vi "Parse Policy.vi"(11 "Response body":string) -> (3 "Policy":T1)   [LabVIEW 2015, in "NI_AWS_IAM.lvlib"]
uses:
  NI_AWS_IAM.lvlib
  Policy.ctl
  XML Parsing/NI_XML Parsing.lvlib
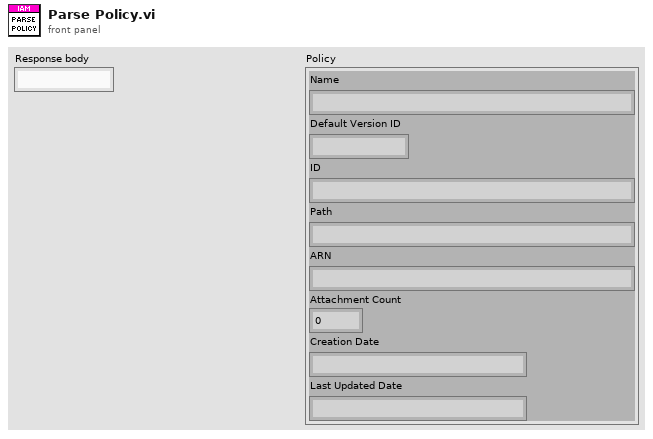
[diagram p1: front panel]
types:
  T1 = typedef "NI_AWS_IAM.lvlib/Policy.ctl" = cluster{"Name":string, "Default Version ID":string, "ID":string, "Path":string, "ARN":string, "Attachment Count":i32, "Creation Date":string, "Last Updated Date":string}
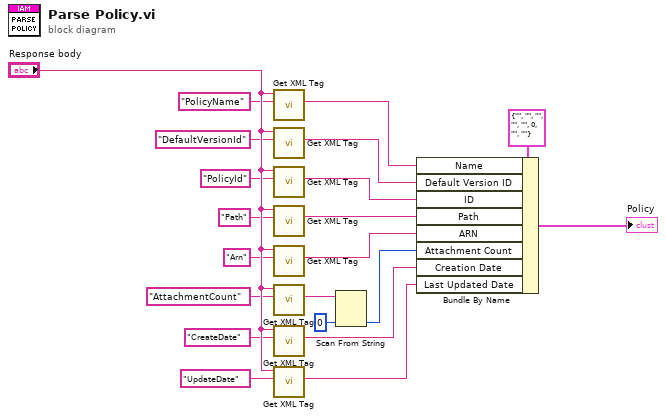
[diagram p0: block diagram]
diagram:
  n1 = call "Get XML Tag.vi"("Tag name"="PolicyName", "XML String in"="Response body") -> ("Tag value"=w10:string)  [unwired: 5 in, 4 out]
  n2 = call "Get XML Tag.vi"("Tag name"="DefaultVersionId", "XML String in"="Response body") -> ("Tag value"=w11:string)  [unwired: 5 in, 4 out]
  n3 = call "Get XML Tag.vi"("Tag name"="PolicyId", "XML String in"="Response body") -> ("Tag value"=w12:string)  [unwired: 5 in, 4 out]
  n4 = call "Get XML Tag.vi"("Tag name"="Path", "XML String in"="Response body") -> ("Tag value"=w13:string)  [unwired: 5 in, 4 out]
  n5 = call "Get XML Tag.vi"("Tag name"="Arn", "XML String in"="Response body") -> ("Tag value"=w14:string)  [unwired: 5 in, 4 out]
  n6 = call "Get XML Tag.vi"("Tag name"="AttachmentCount", "XML String in"="Response body") -> ("Tag value"=w15:string)  [unwired: 5 in, 4 out]
  n7 = call "Get XML Tag.vi"("Tag name"="CreateDate", "XML String in"="Response body") -> ("Tag value"=w18:string)  [unwired: 5 in, 4 out]
  n8 = call "Get XML Tag.vi"("Tag name"="UpdateDate", "XML String in"="Response body") -> ("Tag value"=w21:string)  [unwired: 5 in, 4 out]
  n9 = Scan From String(input string=w15, default 1=0) -> (output 1=w17:i32)  [unwired: 3 in, 3 out]
  n10 = Bundle By Name(cluster=T1 {"Name"="", "Default Version ID"="", "ID"="", "Path"="", "ARN"="", "Attachment Count"=0, "Creation Date"="", "Last Updated Date"=""} ("Policy"), "Name"=w10, "Default Version ID"=w11, "ID"=w12, "Path"=w13, "ARN"=w14, "Attachment Count"=w17, "Creation Date"=w18, "Last Updated Date"=w21) -> (→"Policy":T1)
